vi "6.-Estructura for y Shift Register.vi"() -> ()   [LabVIEW 2020]
panel:
  out "Array":i32[](array[numeric])
  out "element":i32
  out "Waveform Graph":i32[](graph)
  out "x > y?":bool
  out "y":i32
  out "x":i32
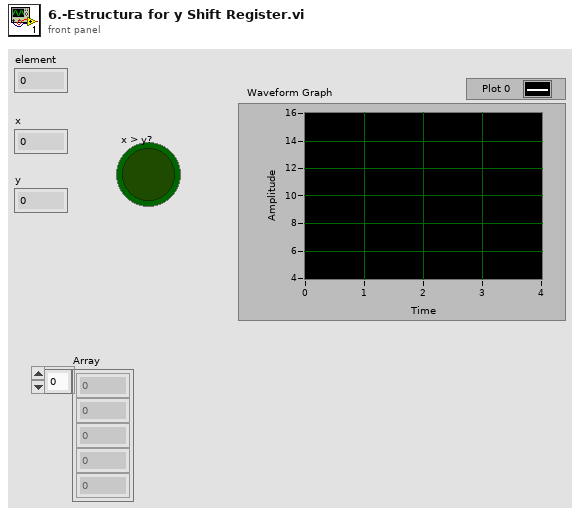
[diagram p1: front panel]
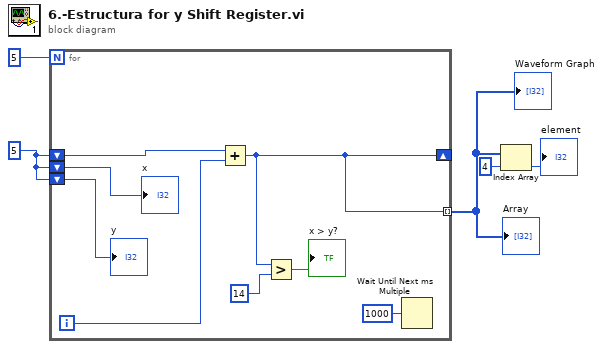
[diagram p0: block diagram]
diagram:
  w4 = 5
  n1 = for {
    N: 5 -> [_]
    shift-right: [w6] -> _
    shift-left: w4 -> [w13]
    shift-left: w4 -> [w11]
    shift-left: w4 -> [w10]
    tunnel: [w6] -> w2 mode=indexing
    i -> [w12]
    n2 = Add(x=w13, y=w12) -> (x+y=w6:i32)
    n3 = Greater?(x=w6, y=14) -> (0:→"x > y?":bool)
    n4 = Wait Until Next ms Multiple(millisecond multiple=u32 1000) -> ()  [unwired: 1 out]
    "x" <- w11
    "y" <- w10
  }
  "Waveform Graph" <- w2
  "Array" <- w2
  n5 = Index Array(array=w2, index=4) -> (element=→"element":i32)
